vi "Mount Public Drive.vi"   [LabVIEW 2012]
uses:
  Anemometry Sub Vis/Globals/Constants_global.vi
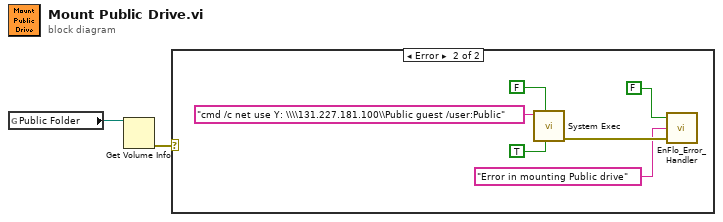
[diagram p0: block diagram]
diagram:
  n1 = global read "Constants_global.vi" "Public Folder"() -> (w2:path)
  n2 = Get Volume Info(11:w2) -> (0:w1:errorcluster)  [unwired: 1 in, 5 out]
  n3 = case shown="Error" w1 {
    frame No Error {
    }
    frame Error {
      n4 = call <vilib>:"System Exec.vi"("run minimized? (F)"=TRUE, "wait until completion? (T)"=FALSE, "command line"="cmd /c net use Y: \\\\131.227.181.100\\Public guest /user:Public") -> ("error out"=w5:errorcluster)  [unwired: 5 in, 3 out]
      n5 = call "EnFlo_Error_Handler.vi"("error in (no error)"=w5, "Error Type"="Error in mounting Public drive", "Dialog Box (T)"=FALSE) -> ()  [unwired: 3 out]
    }
  }
